vi "Update Mode.vi"   [LabVIEW 2014, in "MCP23S17.lvlib"]
doc: "Updates the mode of the pins."
uses:
  MCP23S17.lvlib
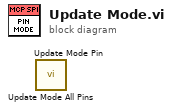
[diagram p0: block diagram]
diagram:
  n1 = call "Update Mode All Pins.vi"() -> ()  [unwired: 9 in, 3 out]
  n2 = call "Update Mode Pin.vi"() -> ()  [unwired: 9 in, 3 out]
